vi "Unary Operation.vi"(4 "Function":u8(ring) items=["bitwise_not", "copy"], 5 "Error":string, 6 "Output Image":T1={"Image ID"=0, "Channel ID"=-1}, 8 "Input Image":T1={"Image ID"=0, "Channel ID"=-1}) -> (0 "Error":string, 1 "Output Image":T1={"Image ID"=0, "Channel ID"=-1}, 3 "Input Image":T1={"Image ID"=0, "Channel ID"=-1})   [LabVIEW 2011, in "labvvis.lvlib"]
uses:
  <userlib>/labvvis/labvvis.lvlib
  <userlib>/labvvis/VVIS Image.ctl
  labvvis.framework
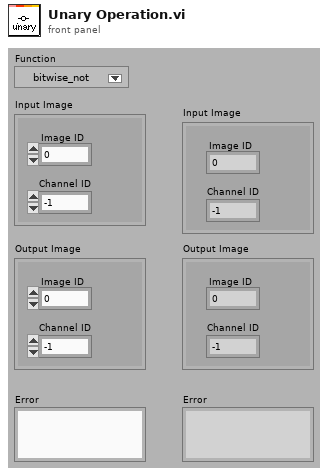
[diagram p1: front panel]
types:
  T1 = typedef "labvvis.lvlib/VVIS Image.ctl" = cluster{"Image ID":i16, "Channel ID":i16}
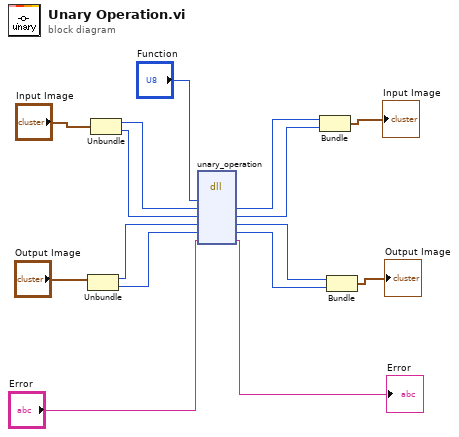
[diagram p0: block diagram]
diagram:
  n1 = Unbundle("Output Image") -> ("Image ID"=w9:i16, "Channel ID"=w8:i16)
  n2 = Unbundle("Input Image") -> ("Image ID"=w13:i16, "Channel ID"=w10:i16)
  n3 = dll-call lib="labvvis.framework" fn="unary_operation"("function"="Function", "src"=w13, "icid"=w10, "out"=w9, "ocid"=w8, "error"="Error") -> ("src"=w12:i16, "icid"=w5:i16, "out"=w4:i16, "ocid"=w3:i16, "error"=→"Error":string)  [unwired: 5 in, 2 out]
  n4 = Bundle("src"=w12, "icid"=w5) -> (→"Input Image":cluster{"src":i16, "icid":i16})  [unwired: 1 in]
  n5 = Bundle("out"=w4, "ocid"=w3) -> (→"Output Image":cluster{"out":i16, "ocid":i16})  [unwired: 1 in]
